vi "2084上传各参数测量周期.vi"(11 "读取各参数测量周期的值":u16[](array[numeric]) caption="读取试剂余量的值") -> (3 "字符串":string)   [LabVIEW 2016, in "数据传输系统.lvlib"]
panel:
  out "数组":cluster{string, "register":u16}[](array[cluster])
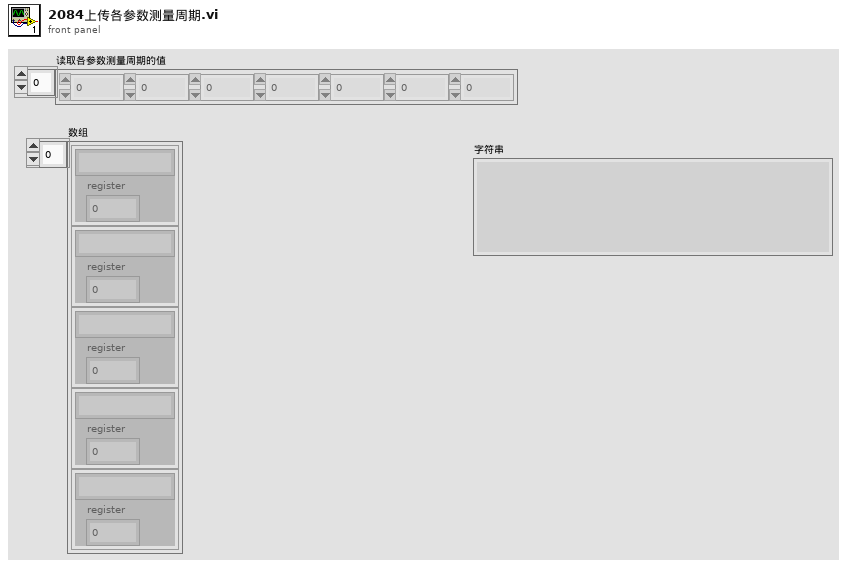
[diagram p1: front panel]
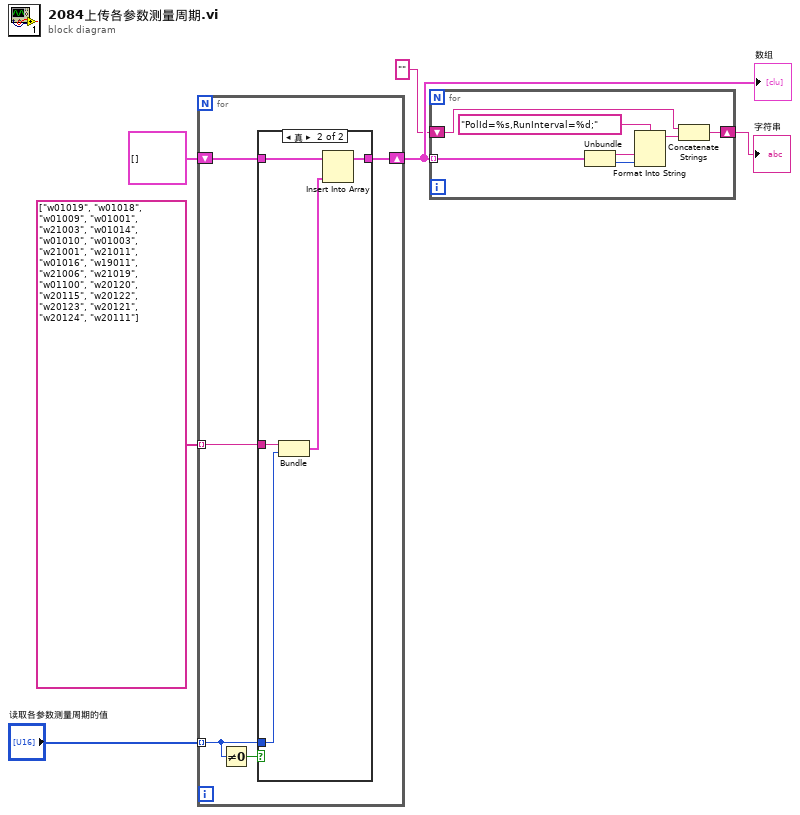
[diagram p0: block diagram]
diagram:
  n1 = for {
    tunnel: "读取各参数测量周期的值" -> [w9] mode=indexing
    tunnel: string[] ["w01019", "w01018", "w01009", "w01001", "w21003", "w01014", "w01010", "w01003", "w21001", "w21011", "w01016", "w19011", "w21006", "w21019", "w01100", "w20120", "w20115", "w20122", "w20123", "w20121", "w20124", "w20111"] -> [w10] mode=indexing
    shift-right: [w7] -> w4
    shift-left: cluster{string, "register":u16}[] [] ("数组") -> [w8]
    n2 = Not Equal To 0?(x=w9) -> (x != 0?=w11:bool)
    n3 = case shown="真" w11 {
      tunnel: w10 -> [_ w16]
      tunnel: w8 -> [w12 w15]
      tunnel: [w12 w13] -> w7
      tunnel: w9 -> [_ w17]
      frame False {
      }
      frame True {
        n4 = Bundle(w16, "register"=w17) -> (w14:cluster{string, "register":u16})  [unwired: 1 in]
        n5 = Insert Into Array(array=w15, new element=w14) -> (w13:cluster{string, "register":u16}[])  [unwired: 1 in]
      }
    }
  }
  "数组" <- w4
  n6 = for {
    tunnel: w4 -> [w23] mode=indexing
    shift-right: [w18] -> w2
    shift-left: "" -> [w19]
    n7 = Unbundle(w23) -> (w22:string, "register"=w21:u16)
    n8 = Format Into String(format string="PolId=%s,RunInterval=%d;", w22, w21) -> (resulting string=w20:string)  [unwired: 2 in, 1 out]
    n9 = Concatenate Strings(w19, w20) -> (w18:string)
  }
  "字符串" <- w2
